vi "stop.vi"(3 "error in (no error)":errorcluster, 4 "stop":bool, 5 "K2602 in":refnum<class "K2602.lvclass">) -> (0 "error out":errorcluster, 1 "Stopped":bool, 2 "K2602 out":refnum<class "K2602.lvclass">)   [LabVIEW 2009, in "Hardware.lvlib" / "Channels.lvlib" / "K2602.lvclass"]
doc: "Abstract Method.\n\nStops the analog output. This vi indicates of the analog output has stopped, and can be used to actively stop the output."
uses:
  K2602.lvclass
  K2602.lvclass/K2602.ctl
  <instrlib>/Keithley 2600 Series/Keithley 2600 Series.lvlib
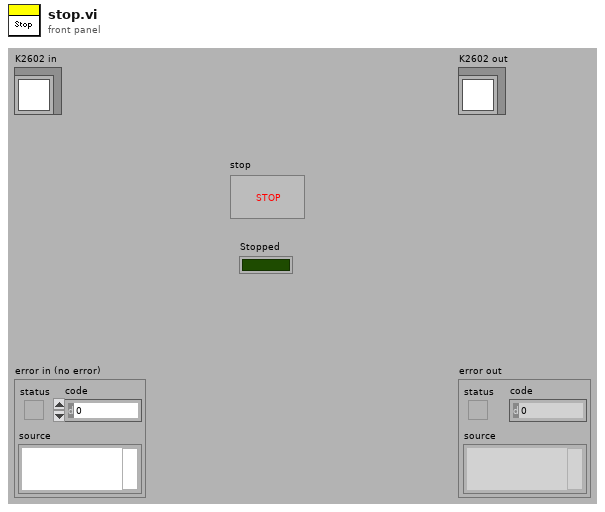
[diagram p1: front panel]
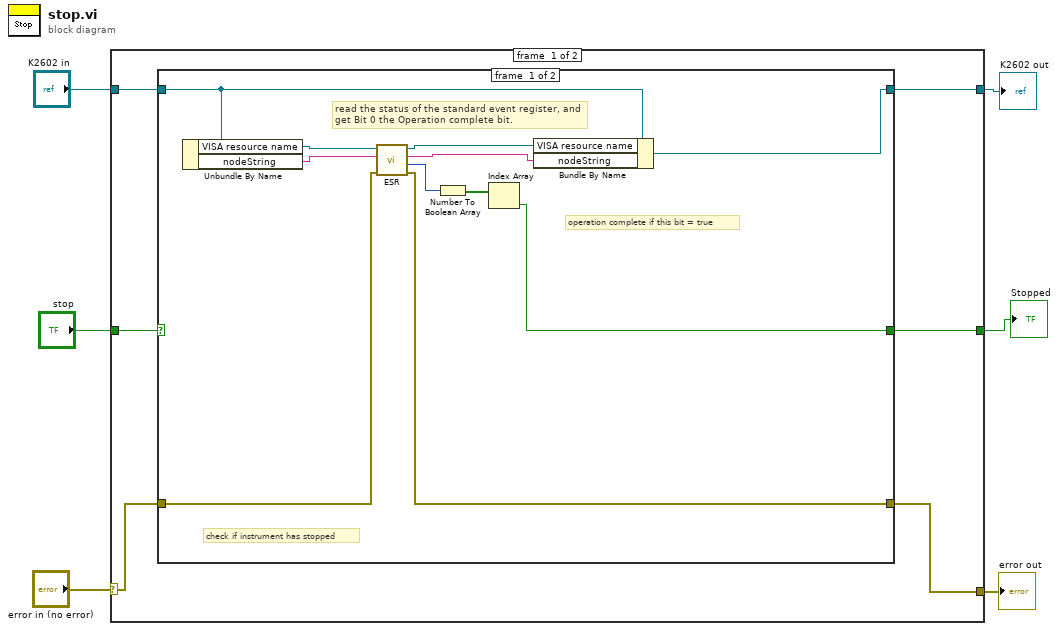
[diagram p0: block diagram]
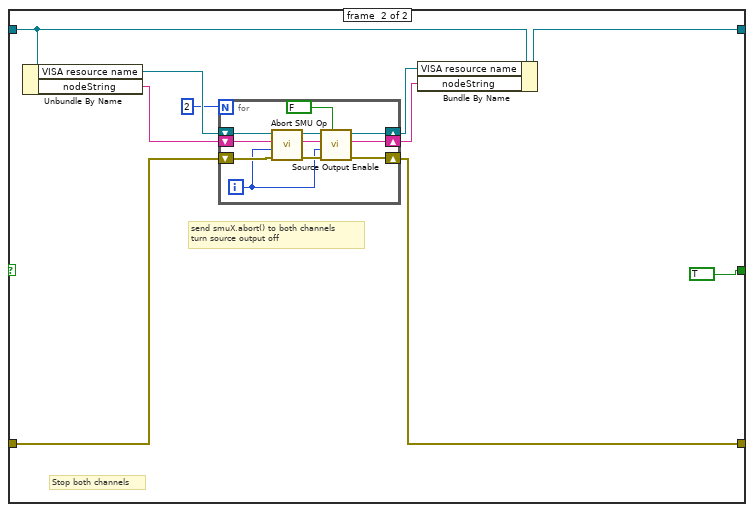
[diagram p2: hidden frame]
diagram:
  n1 = case shown="No Error" "error in (no error)" {
    selector: "error in (no error)" -> [w11 w46]
    tunnel: [w8 w45] -> w5
    tunnel: "K2602 in" -> [w7 w45]
    tunnel: "stop" -> [w12 _]
    tunnel: [w10 w46] -> w2
    tunnel: [w9 _] -> w1
    frame #0 {
      n2 = case shown="True" w12 {
        tunnel: w11 -> [w21 w31]
        tunnel: [w19 w29] -> w10
        tunnel: [w13 TRUE] -> w9
        tunnel: [w18 w26] -> w8
        tunnel: w7 -> [w17 w27]
        frame #0 {
          # "operation complete if this bit = true"
          # "read the status of the standard event register, and \nget Bit 0 the Operation complete bit."
          # "check if instrument has stopped"
          n3 = Unbundle By Name(w17) -> ("VISA resource name"=w23:refnum<visa-resource-name>, "nodeString"=w22:string)
          n4 = call <instrlib>:"ESR.vi"("error in (no error)"=w21, "Node In"=w22, "VISA resource name"=w23) -> ("error out"=w19:errorcluster, "ESR"=w20:u8, "Node Out"=w15:string, "VISA resource name out"=w16:refnum<visa-resource-name>)  [unwired: 4 in, 1 out]
          n5 = Number To Boolean Array(number=w20) -> (Boolean array=w14:bool[])
          n6 = Index Array(array=w14) -> (element=w13:bool)  [unwired: 1 in]
          n7 = Bundle By Name(cluster=w17, "VISA resource name"=w16, "nodeString"=w15) -> (w18:refnum<class "K2602.lvclass">)
        }
        frame #1 {
          # "Stop both channels"
          # "send smuX.abort() to both channels\nturn source output off"
          n8 = Unbundle By Name(w27) -> ("VISA resource name"=w33:refnum<visa-resource-name>, "nodeString"=w32:string)
          n9 = for {
            N: 2 -> [_]
            shift-right: [w36] -> w28
            shift-left: w33 -> [w44]
            shift-right: [w35] -> w25
            shift-left: w32 -> [w43]
            shift-right: [w34] -> w29
            shift-left: w31 -> [w42]
            i -> [w38]
            n10 = call <instrlib>:"Abort SMU Op.vi"("error in"=w42, "Channel (Channel A)"=w38, "Node In"=w43, "VISA resource name"=w44) -> ("error out"=w41:errorcluster, "Node Out"=w40:string, "VISA resource name out"=w39:refnum<visa-resource-name>)  [unwired: 4 in, 1 out]
            n11 = call <instrlib>:"Source Output Enable.vi"("Output (Off)"=FALSE, "error in (no error)"=w41, "Channel (Channel A)"=w38, "Node In"=w40, "VISA resource name"=w39) -> ("error out"=w34:errorcluster, "Node Out"=w35:string, "VISA resource name out"=w36:refnum<visa-resource-name>)  [unwired: 3 in, 1 out]
          }
          n12 = Bundle By Name(cluster=w27, "VISA resource name"=w28, "nodeString"=w25) -> (w26:refnum<class "K2602.lvclass">)
        }
      }
    }
    frame #1 {
    }
  }
  "error out" <- w2
  "K2602 out" <- w5
  "Stopped" <- w1
